vi "S4GUI_003.vi"(7 "Tab ObsEng":enum32{"Obs", "CCD modes", "Guider", "Eng"}(tab)) -> ()   [LabVIEW 2018] (continued)
                        }
                      }
                      frame 3 {
                        n312 = case shown="False" w628 {
                          tunnel: [cluster{u32, u32}[] [{7563008, 7563008}, {7563008, 7563008}] ("Colors [4]") cluster{u32, u32}[] [{16318208, 16318208}, {16318208, 16318208}] ("Colors [4]")] -> w627
                          frame False {
                          }
                          frame True {
                          }
                        }
                        n313 = Not(x=w628) -> (.not. x?=w629:bool)
                      }
                    }
                    "CALW Status" <- w603
                    "PCS" <- w603
                    n314 = property on="CALW Status" class="Bool (strict)"("Colors [4]"=w601) -> ()  [unwired: 2 in, 2 out]
                    n315 = property on="PCS" class="Bool (strict)"("Colors [4]"=w601, "BoolText.Text"=w602) -> ()  [unwired: 2 in, 2 out]
                  }
                  frame #3 {
                    # "ASEL"
                    n316 = Unbundle By Name(w641) -> ("ASEL State"=w640:i32)
                    n317 = Unbundle By Name(w637) -> ("ASEL posname"=w634:string)
                    n318 = local read "ASEL Status"() -> (w635:bool)
                    n319 = case shown="Default" w634 {
                      selector: w634 -> [w642 _ _]
                      tunnel: [w642 "OFF" ("y") "ON" ("y")] -> w633
                      frame Default {
                      }
                      frame "OFF" {
                      }
                      frame "ON" {
                      }
                    }
                    n320 = case shown="3" w640 {
                      tunnel: [cluster{u32, u32}[] [{9868950, 9868950}, {9868950, 9868950}] ("Colors [4]") cluster{u32, u32}[] [{9868950, 9868950}, {9868950, 9868950}] ("Colors [4]") cluster{u32, u32}[] [{16318208, 16318208}, {16318208, 16318208}] ("Colors [4]") cluster{u32, u32}[] [{6618880, 6618880}, {6618880, 6618880}] ("Colors [4]") w660] -> w638
                      tunnel: [FALSE ("WPROT Status") FALSE ("WPROT Status") TRUE FALSE ("WPROT Status") w659] -> w639
                      tunnel: w633 -> [_ _ _ w655 _]
                      tunnel: ["" ("y") "" ("y") "" ("y") w655 "" ("y")] -> w636
                      tunnel: w635 -> [_ _ _ _ w657]
                      frame Default {
                      }
                      frame 0 {
                      }
                      frame 1 {
                      }
                      frame 2 {
                      }
                      frame 3 {
                        n321 = case shown="True" w657 {
                          tunnel: [cluster{u32, u32}[] [{7563008, 7563008}, {7563008, 7563008}] ("Colors [4]") cluster{u32, u32}[] [{16318208, 16318208}, {16318208, 16318208}] ("Colors [4]")] -> w660
                          frame False {
                          }
                          frame True {
                          }
                        }
                        n322 = Not(x=w657) -> (.not. x?=w659:bool)
                      }
                    }
                    "ASEL Status" <- w639
                    "Analyzer" <- w639
                    n323 = property on="Analyzer" class="Bool (strict)"("Colors [4]"=w638, "BoolText.Text"=w636) -> ()  [unwired: 2 in, 2 out]
                    n324 = property on="ASEL Status" class="Bool (strict)"("Colors [4]"=w638) -> ()  [unwired: 2 in, 2 out]
                  }
                  frame #4 {
                    # "GMIR & GFOC"
                    n325 = Unbundle By Name(w670) -> ("GMIR State"=w669:i32, "GFOC State"=w668:i32)
                    n326 = case shown="2" w669 {
                      tunnel: [cluster{u32, u32}[] [{9868950, 9868950}, {9868950, 9868950}] ("Colors [4]") cluster{u32, u32}[] [{9868950, 9868950}, {9868950, 9868950}] ("Colors [4]") cluster{u32, u32}[] [{16318208, 16318208}, {16318208, 16318208}] ("Colors [4]") cluster{u32, u32}[] [{6618880, 6618880}, {6618880, 6618880}] ("Colors [4]") cluster{u32, u32}[] [{16318208, 16318208}, {16318208, 16318208}] ("Colors [4]")] -> w663
                      tunnel: [FALSE ("WPROT Status") FALSE ("WPROT Status") TRUE ("WPROT Status") FALSE ("WPROT Status") TRUE ("WPROT Status")] -> w665
                      frame Default {
                      }
                      frame 0 {
                      }
                      frame 1 {
                      }
                      frame 2 {
                      }
                      frame 3 {
                      }
                    }
                    "GMIR Status" <- w665
                    "GMIR Status 2" <- w665
                    n327 = property on="GMIR Status" class="Bool (strict)"("Colors [4]"=w663) -> ()  [unwired: 2 in, 2 out]
                    n328 = property on="GMIR Status 2" class="Bool (strict)"("Colors [4]"=w663) -> ()  [unwired: 2 in, 2 out]
                    n329 = case shown="Default" w668 {
                      tunnel: [cluster{u32, u32}[] [{9868950, 9868950}, {9868950, 9868950}] ("Colors [4]") cluster{u32, u32}[] [{9868950, 9868950}, {9868950, 9868950}] ("Colors [4]") cluster{u32, u32}[] [{16318208, 16318208}, {16318208, 16318208}] ("Colors [4]") cluster{u32, u32}[] [{6618880, 6618880}, {6618880, 6618880}] ("Colors [4]") cluster{u32, u32}[] [{16318208, 16318208}, {16318208, 16318208}] ("Colors [4]")] -> w664
                      tunnel: [FALSE ("WPROT Status") FALSE ("WPROT Status") TRUE ("WPROT Status") FALSE ("WPROT Status") TRUE ("WPROT Status")] -> w666
                      frame Default {
                      }
                      frame 0 {
                      }
                      frame 1 {
                      }
                      frame 2 {
                      }
                      frame 3 {
                      }
                    }
                    "GFOC Status" <- w666
                    "GFOC Status 2" <- w666
                    n330 = Or(x=w665, y=w666) -> (x .or. y?=w667:bool)
                    n331 = property on="GFOC Status" class="Bool (strict)"("Colors [4]"=w664) -> ()  [unwired: 2 in, 2 out]
                    n332 = property on="GFOC Status 2" class="Bool (strict)"("Colors [4]"=w664) -> ()  [unwired: 2 in, 2 out]
                    n333 = property on="GS led" class="Bool (strict)"("Blinking"=w667, "Value"=w667) -> ()  [unwired: 2 in, 2 out]
                  }
                }
              }
              frame #7 {
                n334 = Unbundle By Name(w693) -> ("Instrument Pos Names"=w692:T21)
                n335 = stacked-sequence {
                  tunnel: w692 -> [w695 w712 w737 w763]
                  tunnel: [_ _ _ w764] -> w691
                  frame #0 {
                    n336 = Unbundle By Name(w695) -> ("WPSEL posname"=w694:string)
                    n337 = case shown="\"L/2\", \"L/4\", \"OFF\"" w694 {
                      selector: w694 -> [_ w696]
                      frame "False", Default {
                      }
                      frame "L/2", "L/4", "OFF" {
                        n338 = First Call?() -> (First Call?: T/F=w697:bool)
                        n339 = case shown="True" w697 {
                          tunnel: w696 -> [_ w698]
                          frame False {
                          }
                          frame True {
                            n340 = case shown="\"False\", Default" w698 {
                              frame "False", Default {
                              }
                              frame "L/2" {
                                w699 = u16 1 items=["OFF", "Lambda/2", "Lambda/4"] ("Lambda Selector")
                                n341 = property on="Lambda Selector" class="Ring (strict)"(error in=errorcluster {"status"=FALSE, "code"=0, "source"=""} ("error in (no error)"), "Value"=w699) -> (error out=w701:errorcluster)  [unwired: 1 in, 1 out]
                                n342 = property on="Lambda Selector" class="Ring (strict)"(error in=w701, "RingText.Text"="Lambda/2" ("Boolean Text.Text")) -> ()  [unwired: 1 in, 2 out]
                              }
                              frame "L/4" {
                                w703 = u16 2 items=["OFF", "Lambda/2", "Lambda/4"] ("Lambda Selector")
                                n343 = property on="Lambda Selector" class="Ring (strict)"(error in=errorcluster {"status"=FALSE, "code"=0, "source"=""} ("error in (no error)"), "Value"=w703) -> (error out=w705:errorcluster)  [unwired: 1 in, 1 out]
                                n344 = property on="Lambda Selector" class="Ring (strict)"(error in=w705, "RingText.Text"="Lambda/4" ("Boolean Text.Text")) -> ()  [unwired: 1 in, 2 out]
                              }
                              frame "OFF" {
                                w708 = u16 0 items=["OFF", "Lambda/2", "Lambda/4"] ("Lambda Selector")
                                (unwired) "Select..." ("Boolean Text.Text")
                                n345 = property on="Lambda Selector" class="Ring (strict)"(error in=errorcluster {"status"=FALSE, "code"=0, "source"=""} ("error in (no error)"), "Value"=w708) -> (error out=w710:errorcluster)  [unwired: 1 in, 1 out]
                                n346 = property on="Lambda Selector" class="Ring (strict)"(error in=w710, "RingText.Text"="OFF" ("Boolean Text.Text")) -> ()  [unwired: 1 in, 2 out]
                              }
                            }
                          }
                        }
                      }
                    }
                  }
                  frame #1 {
                    n347 = Unbundle By Name(w712) -> ("CALW posname"=w711:string)
                    n348 = case shown="\"DEPOLARIZER\", \"OFF\", \"PINHOLE\", \"POLARIZER\", \"SHUTTER\"" w711 {
                      selector: w711 -> [_ w713]
                      frame "False", Default {
                      }
                      frame "DEPOLARIZER", "OFF", "PINHOLE", "POLARIZER", "SHUTTER" {
                        n349 = First Call?() -> (First Call?: T/F=w714:bool)
                        n350 = case shown="True" w714 {
                          tunnel: w713 -> [_ w715]
                          frame False {
                          }
                          frame True {
                            n351 = case shown="\"OFF\"" w715 {
                              frame "False", Default {
                              }
                              frame "POLARIZER" {
                                w716 = u16 1 items=["OFF", "POLARIZER", "PINHOLE", "SHUTTER", "DEPOLARIZER"] ("Calibrator Selector")
                                n352 = property on="Calibrator Selector" class="Ring (strict)"(error in=errorcluster {"status"=FALSE, "code"=0, "source"=""} ("error in (no error)"), "Value"=w716) -> (error out=w718:errorcluster)  [unwired: 1 in, 1 out]
                                n353 = property on="Calibrator Selector" class="Ring (strict)"(error in=w718, "RingText.Text"="POLARIZER" ("Boolean Text.Text")) -> ()  [unwired: 1 in, 2 out]
                              }
                              frame "DEPOLARIZER" {
                                w720 = u16 4 items=["OFF", "POLARIZER", "PINHOLE", "SHUTTER", "DEPOLARIZER"] ("Calibrator Selector")
                                n354 = property on="Calibrator Selector" class="Ring (strict)"(error in=errorcluster {"status"=FALSE, "code"=0, "source"=""} ("error in (no error)"), "Value"=w720) -> (error out=w722:errorcluster)  [unwired: 1 in, 1 out]
                                n355 = property on="Calibrator Selector" class="Ring (strict)"(error in=w722, "RingText.Text"="DEPOLARIZER" ("Boolean Text.Text")) -> ()  [unwired: 1 in, 2 out]
                              }
                              frame "PINHOLE" {
                                w724 = u16 2 items=["OFF", "POLARIZER", "PINHOLE", "SHUTTER", "DEPOLARIZER"] ("Calibrator Selector")
                                n356 = property on="Calibrator Selector" class="Ring (strict)"(error in=errorcluster {"status"=FALSE, "code"=0, "source"=""} ("error in (no error)"), "Value"=w724) -> (error out=w726:errorcluster)  [unwired: 1 in, 1 out]
                                n357 = property on="Calibrator Selector" class="Ring (strict)"(error in=w726, "RingText.Text"="PINHOLE" ("Boolean Text.Text")) -> ()  [unwired: 1 in, 2 out]
                              }
                              frame "SHUTTER" {
                                w728 = u16 3 items=["OFF", "POLARIZER", "PINHOLE", "SHUTTER", "DEPOLARIZER"] ("Calibrator Selector")
                                n358 = property on="Calibrator Selector" class="Ring (strict)"(error in=errorcluster {"status"=FALSE, "code"=0, "source"=""} ("error in (no error)"), "Value"=w728) -> (error out=w730:errorcluster)  [unwired: 1 in, 1 out]
                                n359 = property on="Calibrator Selector" class="Ring (strict)"(error in=w730, "RingText.Text"="SHUTTER" ("Boolean Text.Text")) -> ()  [unwired: 1 in, 2 out]
                              }
                              frame "OFF" {
                                w732 = u16 0 items=["OFF", "POLARIZER", "PINHOLE", "SHUTTER", "DEPOLARIZER"] ("Calibrator Selector")
                                n360 = property on="Calibrator Selector" class="Ring (strict)"(error in=errorcluster {"status"=FALSE, "code"=0, "source"=""} ("error in (no error)"), "Value"=w732) -> (error out=w734:errorcluster)  [unwired: 1 in, 1 out]
                                n361 = property on="Calibrator Selector" class="Ring (strict)"(error in=w734, "RingText.Text"="OFF" ("Boolean Text.Text")) -> ()  [unwired: 1 in, 2 out]
                              }
                            }
                          }
                        }
                      }
                    }
                  }
                  frame #2 {
                    n362 = Unbundle By Name(w737) -> ("WPROT posname"=w736:string)
                    "Name" <- w736
                    n363 = stacked-sequence {
                      tunnel: w736 -> [_ w739]
                      frame #0 {
                        w738 = FALSE
                        "ledP0" <- w738
                        "ledP1" <- w738
                        "ledP2" <- w738
                        "ledP3" <- w738
                        "ledP4" <- w738
                        "ledP5" <- w738
                        "ledP6" <- w738
                        "ledP7" <- w738
                        "ledP8" <- w738
                        "ledP9" <- w738
                        "ledP10" <- w738
                        "ledP11" <- w738
                        "ledP12" <- w738
                        "ledP13" <- w738
                        "ledP14" <- w738
                        "ledP15" <- w738
                      }
                      frame #1 {
                        n364 = case shown="\"WP3\"" w739 {
                          frame Default {
                          }
                          frame "WP1" {
                            n365 = local write "ledP0"(TRUE ("ledP0")) -> ()
                          }
                          frame "WP2" {
                            n366 = local write "ledP1"(TRUE ("ledP0")) -> ()
                          }
                          frame "WP3" {
                            n367 = local write "ledP2"(TRUE ("ledP0")) -> ()
                          }
                          frame "WP4" {
                            n368 = local write "ledP3"(TRUE ("ledP0")) -> ()
                          }
                          frame "WP5" {
                            n369 = local write "ledP4"(TRUE ("ledP0")) -> ()
                          }
                          frame "WP6" {
                            n370 = local write "ledP5"(TRUE ("ledP0")) -> ()
                          }
                          frame "WP7" {
                            n371 = local write "ledP6"(TRUE ("ledP0")) -> ()
                          }
                          frame "WP8" {
                            n372 = local write "ledP7"(TRUE ("ledP0")) -> ()
                          }
                          frame "WP9" {
                            n373 = local write "ledP8"(TRUE ("ledP0")) -> ()
                          }
                          frame "WP10" {
                            n374 = local write "ledP9"(TRUE ("ledP0")) -> ()
                          }
                          frame "WP11" {
                            n375 = local write "ledP10"(TRUE ("ledP0")) -> ()
                          }
                          frame "WP12" {
                            n376 = local write "ledP11"(TRUE ("ledP0")) -> ()
                          }
                          frame "WP13" {
                            n377 = local write "ledP12"(TRUE ("ledP0")) -> ()
                          }
                          frame "WP14" {
                            n378 = local write "ledP13"(TRUE ("ledP0")) -> ()
                          }
                          frame "WP15" {
                            n379 = local write "ledP14"(TRUE ("ledP0")) -> ()
                          }
                          frame "WP16" {
                            n380 = local write "ledP15"(TRUE ("ledP0")) -> ()
                          }
                        }
                      }
                    }
                  }
                  frame #3 {
                    w767 = "OFF" ("Boolean Text.Text")
                    # "Polarimetria:   ASEL = ON  &   (WPSEL =L/2 or L/4)\n\nFotometria:    ASEL=OFF & WPSEL = OFF & CALW = OFF"
                    n381 = Unbundle By Name(w763) -> ("ASEL posname"=w758:string, "WPSEL posname"=w760:string, "CALW posname"=w759:string)
                    n382 = Unbundle By Name(w763) -> ("WPSEL posname"=w770:string, "CALW posname"=w771:string, "ASEL posname"=w765:string)
                    n383 = Equal?(x=w758, y="ON" ("Boolean Text.Text")) -> (x = y?=w761:bool)
                    n384 = case shown="True" w761 {
                      tunnel: w760 -> [w780 w789]
                      tunnel: w759 -> [w779 w783]
                      tunnel: w758 -> [w776 _]
                      tunnel: [FALSE ("Polarimetric Mode") w784] -> w757
                      tunnel: [w772 FALSE ("Photometric Mode")] -> w756
                      frame False {
                        w775 = "OFF" ("Boolean Text.Text")
                        n385 = Equal?(x=w776, y=w775) -> (x = y?=w774:bool)
                        n386 = Equal?(x=w779, y=w775) -> (x = y?=w777:bool)
                        n387 = Equal?(x=w780, y=w775) -> (x = y?=w778:bool)
                        n388 = Compound Arithmetic op=AND(w774, w778, w777) -> (w772:bool)
                      }
                      frame True {
                        n389 = Equal?(x="L/2" ("Boolean Text.Text"), y=w789) -> (x = y?=w790:bool)
                        n390 = Equal?(x="L/4" ("Boolean Text.Text"), y=w789) -> (x = y?=w787:bool)
                        n391 = Not Equal?(x="SHUTTER", y=w783) -> (x != y?=w781:bool)
                        n392 = Or(x=w790, y=w787) -> (x .or. y?=w785:bool)
                        n393 = And(x=w785, y=w781) -> (x .and. y?=w784:bool)
                      }
                    }
                    "Polarimetric Mode" <- w757
                    "Photometric Mode" <- w756
                    n394 = Equal?(x=w767, y=w770) -> (x = y?=w768:bool)
                    n395 = Equal?(x=w767, y=w771) -> (x = y?=w769:bool)
                    n396 = Equal?(x=w767, y=w765) -> (x = y?=w766:bool)
                    n397 = Compound Arithmetic op=AND(w768, w769, w766) -> (invert w764:bool)
                  }
                }
              }
              frame #8 {
                n398 = Unbundle By Name(w796) -> ("ChannelA_Status"=w795:T22, "ChannelB_Status"=w794:T22, "ChannelC_Status"=w792:T22, "ChannelD_Status"=w793:T22)
                n399 = stacked-sequence {
                  tunnel: w795 -> [w884 w940 w992 w1069 _ _ _]
                  tunnel: w794 -> [w883 w938 w991 _ w1090 _ _]
                  tunnel: w793 -> [w881 w935 w989 _ _ _ w1132]
                  tunnel: w792 -> [w882 w936 w990 _ _ w1111 _]
                  frame #0 {
                    n400 = Unbundle By Name(w881) -> ("connection"=w861:bool, "FT"=w843:bool, "Current exp"=w820:dbl, "Cooler ON/OFF"=w875:i16, "Currently temperature"=w872:i16, "Temperature Status"=w869:string, "target  temp"=w805:i16)
                    "Exposure Time ch4" <- w820
                    n401 = Unbundle By Name(w883) -> ("connection"=w863:bool, "FT"=w847:bool, "Current exp"=w831:dbl, "Cooler ON/OFF"=w877:i16, "Currently temperature"=w874:i16, "Temperature Status"=w871:string, "target  temp"=w809:i16)
                    "Exposure Time ch2" <- w831
                    n402 = Unbundle By Name(w884) -> ("connection"=w864:bool, "FT"=w848:bool, "Current exp"=w840:dbl, "Cooler ON/OFF"=w880:i16, "Currently temperature"=w878:i16, "Temperature Status"=w879:string, "target  temp"=w817:i16)
                    "Exposure Time ch1" <- w840
                    n403 = Unbundle By Name(w882) -> ("connection"=w862:bool, "FT"=w845:bool, "Current exp"=w821:dbl, "Cooler ON/OFF"=w876:i16, "Currently temperature"=w873:i16, "Temperature Status"=w870:string, "target  temp"=w806:i16)
                    "Exposure Time ch3" <- w821
                    n404 = Number To Decimal String(number=w805) -> (decimal integer string=→"Target Temp 4":string)  [unwired: 1 in]
                    n405 = Number To Decimal String(number=w806) -> (decimal integer string=→"Target Temp 3":string)  [unwired: 1 in]
                    n406 = Number To Decimal String(number=w809) -> (decimal integer string=→"Target Temp 2":string)  [unwired: 1 in]
                    n407 = Not Equal To 0?(x=w875) -> (x != 0?=w866:bool)
                    n408 = First Call?() -> (First Call?: T/F=w858:bool)
                    n409 = First Call?() -> (First Call?: T/F=w860:bool)
                    n410 = First Call?() -> (First Call?: T/F=w857:bool)
                    n411 = Not Equal To 0?(x=w876) -> (x != 0?=w865:bool)
                    n412 = First Call?() -> (First Call?: T/F=w859:bool)
                    n413 = Number To Decimal String(number=w817) -> (decimal integer string=→"Target Temp 1":string)  [unwired: 1 in]
                    n414 = Number To Fractional String(use system decimal point (T)=FALSE, number=w840, precision (6)=i16 2) -> (F-format string=w837:string)  [unwired: 1 in]
                    n415 = case shown="True" w858 {
                      tunnel: w806 -> [_ w886]
                      frame False {
                      }
                      frame True {
                        n416 = property on="Target Temp 3" class="DigNum (strict)"("Value"=w886) -> ()  [unwired: 2 in, 2 out]
                      }
                    }
                    n417 = case shown="True" w860 {
                      tunnel: w817 -> [_ w888]
                      frame False {
                      }
                      frame True {
                        n418 = property on="Target Temp 1" class="DigNum (strict)"("Value"=w888) -> ()  [unwired: 2 in, 2 out]
                      }
                    }
                    n419 = Number To Fractional String(use system decimal point (T)=FALSE, number=w831, precision (6)=i16 2) -> (F-format string=w832:string)  [unwired: 1 in]
                    n420 = case shown="True" w857 {
                      tunnel: w805 -> [_ w885]
                      frame False {
                      }
                      frame True {
                        n421 = property on="Target Temp 4" class="DigNum (strict)"("Value"=w885) -> ()  [unwired: 2 in, 2 out]
                      }
                    }
                    n422 = Concatenate Strings("Exposure Time ", w837) -> (w836:string)
                    n423 = Number To Fractional String(use system decimal point (T)=FALSE, number=w821, precision (6)=i16 2) -> (F-format string=w822:string)  [unwired: 1 in]
                    n424 = Number To Fractional String(use system decimal point (T)=FALSE, number=w820, precision (6)=i16 2) -> (F-format string=w826:string)  [unwired: 1 in]
                    n425 = Concatenate Strings("Exposure Time ", w832) -> (w830:string)
                    n426 = case shown="True" w859 {
                      tunnel: w809 -> [_ w887]
                      frame False {
                      }
                      frame True {
                        n427 = property on="Target Temp 2" class="DigNum (strict)"("Value"=w887) -> ()  [unwired: 2 in, 2 out]
                      }
                    }
                    n428 = Concatenate Strings("Exposure Time ", w822) -> (w818:string)
                    n429 = Concatenate Strings("Exposure Time ", w826) -> (w819:string)
                    n430 = property on="Exposure Time ch1" class="Slide (strict)"("Caption.Text"=w836) -> ()  [unwired: 2 in, 2 out]
                    n431 = property on="Exposure Time ch2" class="Slide (strict)"("Caption.Text"=w830) -> ()  [unwired: 2 in, 2 out]
                    n432 = property on="Exposure Time ch3" class="Slide (strict)"("Caption.Text"=w818) -> ()  [unwired: 2 in, 2 out]
                    n433 = property on="Exposure Time ch4" class="Slide (strict)"("Caption.Text"=w819) -> ()  [unwired: 2 in, 2 out]
                    n434 = Not Equal To 0?(x=w880) -> (x != 0?=w867:bool)
                    n435 = Not Equal To 0?(x=w877) -> (x != 0?=w868:bool)
                    n436 = case shown="True" w864 {
                      tunnel: w879 -> [_ w919]
                      tunnel: w878 -> [_ w920]
                      tunnel: w867 -> [_ w917]
                      tunnel: [FALSE w917] -> w856
                      tunnel: [i16 0 ("Currently temperature") w920] -> w814
                      tunnel: ["" ("Temperature Status") w919] -> w855
                      tunnel: [FALSE w918] -> w849
                      tunnel: w848 -> [_ w918]
                      frame False {
                      }
                      frame True {
                      }
                    }
                    "Cooler status 1" <- w856
                    "Curr Temp 1" <- w814
                    "Temp Status 1" <- w855
                    "Panel Temp" <- w814
                    "Panel cooler 1" <- w856
                    "FT1" <- w849
                    n437 = case shown="False" w863 {
                      tunnel: w874 -> [_ w911]
                      tunnel: w871 -> [_ w910]
                      tunnel: w868 -> [_ w912]
                      tunnel: [FALSE w912] -> w854
                      tunnel: [i16 0 ("Currently temperature") w911] -> w810
                      tunnel: ["" ("Temperature Status") w910] -> w853
                      tunnel: w847 -> [_ w909]
                      tunnel: [FALSE ("FT") w909] -> w846
                      frame False {
                      }
                      frame True {
                      }
                    }
                    "Panel Temp 2" <- w810
                    "Curr Temp 2" <- w810
                    "Cooler status 2" <- w854
                    "Panel cooler 2" <- w854
                    "Temp Status 2" <- w853
                    "FT2" <- w846
                    n438 = case shown="True" w861 {
                      tunnel: w872 -> [_ w895]
                      tunnel: w869 -> [_ w894]
                      tunnel: w866 -> [_ w896]
                      tunnel: [FALSE w896] -> w851
                      tunnel: [i16 0 ("Currently temperature") w895] -> w798
                      tunnel: ["" ("Temperature Status") w894] -> w850
                      tunnel: w843 -> [_ w893]
                      tunnel: [FALSE ("FT") w893] -> w842
                      frame False {
                      }
                      frame True {
                      }
                    }
                    "Cooler status 4" <- w851
                    "Panel Temp 4" <- w798
                    "Curr Temp 4" <- w798
                    "Temp Status 4" <- w850
                    "Panel cooler 4" <- w851
                    "FT4" <- w842
                    n439 = case shown="True" w862 {
                      tunnel: w873 -> [_ w903]
                      tunnel: w870 -> [_ w902]
                      tunnel: w865 -> [_ w904]
                      tunnel: [FALSE w904] -> w852
                      tunnel: [i16 0 ("Currently temperature") w903] -> w799
                      tunnel: ["" ("Temperature Status") w902] -> w797
                      tunnel: w845 -> [_ w901]
                      tunnel: [FALSE ("FT") w901] -> w844
                      frame False {
                      }
                      frame True {
                      }
                    }
                    "Cooler status 3" <- w852
                    "Panel Temp 3" <- w799
                    "Curr Temp 3" <- w799
                    "Panel cooler 3" <- w852
                    "FT3" <- w844
                    "Temp Status 3" <- w797
                    n440 = Number To Decimal String(number=w810) -> (decimal integer string=w811:string)  [unwired: 1 in]
                    n441 = Number To Decimal String(number=w814) -> (decimal integer string=w815:string)  [unwired: 1 in]
                    n442 = property on="Panel cooler 2" class="Bool (strict)"("BoolText.Text"=w811, "BoolText.Justify"=enum16{"Left", "Center", "Right"}."Right" ("Boolean Text.Justification")) -> ()  [unwired: 2 in, 2 out]
                    n443 = property on="Panel cooler 1" class="Bool (strict)"("BoolText.Text"=w815, "BoolText.Justify"=enum16{"Left", "Center", "Right"}."Right" ("Boolean Text.Justification")) -> ()  [unwired: 2 in, 2 out]
                    n444 = Number To Decimal String(number=w799) -> (decimal integer string=w803:string)  [unwired: 1 in]
                    n445 = Number To Decimal String(number=w798) -> (decimal integer string=w800:string)  [unwired: 1 in]
                    n446 = property on="Panel cooler 3" class="Bool (strict)"("BoolText.Text"=w803, "BoolText.Justify"=enum16{"Left", "Center", "Right"}."Right" ("Boolean Text.Justification")) -> ()  [unwired: 2 in, 2 out]
                    n447 = property on="Panel cooler 4" class="Bool (strict)"("BoolText.Text"=w800, "BoolText.Justify"=enum16{"Left", "Center", "Right"}."Right" ("Boolean Text.Justification")) -> ()  [unwired: 2 in, 2 out]
                  }
                  frame #1 {
                    n448 = Unbundle By Name(w935) -> ("LastFileImage"=→"Last Image ch4":string, "Temperature Status"=w923:string)
                    n449 = Unbundle By Name(w936) -> ("LastFileImage"=→"Last Image ch3":string, "Temperature Status"=w924:string)
                    n450 = Unbundle By Name(w938) -> ("LastFileImage"=→"Last Image ch2":string, "Temperature Status"=w927:string)
                    n451 = Unbundle By Name(w940) -> ("LastFileImage"=→"Last Image ch1":string, "Temperature Status"=w932:string)
                    n452 = case shown="Default" w932 {
                      tunnel: [cluster{u32, u32}[] [{6124107, 6124107}, {6124107, 6124107}] ("Colors [4]") cluster{u32, u32}[] [{6618880, 6618880}, {6618880, 6618880}] ("Colors [4]") cluster{u32, u32}[] [{16318208, 16318208}, {16318208, 16318208}] ("Colors [4]") cluster{u32, u32}[] [{8554752, 8554752}, {8554752, 8554752}] ("Colors [4]")] -> w931
                      tunnel: [FALSE FALSE FALSE TRUE] -> w930
                      frame Default {
                      }
                      frame "TEMPERATURE_STABILIZED" {
                      }
                      frame "TEMPERATURE_NOT_STABILIZED" {
                      }
                      frame "TEMPERATURE_NOT_REACHED" {
                      }
                    }
                    n453 = case shown="\"TEMPERATURE_NOT_REACHED\"" w927 {
                      tunnel: [cluster{u32, u32}[] [{6124107, 6124107}, {6124107, 6124107}] ("Colors [4]") cluster{u32, u32}[] [{6618880, 6618880}, {6618880, 6618880}] ("Colors [4]") cluster{u32, u32}[] [{16318208, 16318208}, {16318208, 16318208}] ("Colors [4]") cluster{u32, u32}[] [{8554752, 8554752}, {8554752, 8554752}] ("Colors [4]")] -> w929
                      tunnel: [FALSE FALSE FALSE TRUE] -> w928
                      frame Default {
                      }
                      frame "TEMPERATURE_STABILIZED" {
                      }
                      frame "TEMPERATURE_NOT_STABILIZED" {
                      }
                      frame "TEMPERATURE_NOT_REACHED" {
                      }
                    }
                    n454 = case shown="\"TEMPERATURE_NOT_REACHED\"" w924 {
                      tunnel: [cluster{u32, u32}[] [{6124107, 6124107}, {6124107, 6124107}] ("Colors [4]") cluster{u32, u32}[] [{6618880, 6618880}, {6618880, 6618880}] ("Colors [4]") cluster{u32, u32}[] [{16318208, 16318208}, {16318208, 16318208}] ("Colors [4]") cluster{u32, u32}[] [{8554752, 8554752}, {8554752, 8554752}] ("Colors [4]")] -> w926
                      tunnel: [FALSE FALSE FALSE TRUE] -> w925
                      frame Default {
                      }
                      frame "TEMPERATURE_STABILIZED" {
                      }
                      frame "TEMPERATURE_NOT_STABILIZED" {
                      }
                      frame "TEMPERATURE_NOT_REACHED" {
                      }
                    }
                    n455 = case shown="\"TEMPERATURE_NOT_REACHED\"" w923 {
                      tunnel: [cluster{u32, u32}[] [{6124107, 6124107}, {6124107, 6124107}] ("Colors [4]") cluster{u32, u32}[] [{6618880, 6618880}, {6618880, 6618880}] ("Colors [4]") cluster{u32, u32}[] [{16318208, 16318208}, {16318208, 16318208}] ("Colors [4]") cluster{u32, u32}[] [{8554752, 8554752}, {8554752, 8554752}] ("Colors [4]")] -> w922
                      tunnel: [FALSE FALSE FALSE TRUE] -> w921
                      frame Default {
                      }
                      frame "TEMPERATURE_STABILIZED" {
                      }
                      frame "TEMPERATURE_NOT_STABILIZED" {
                      }
                      frame "TEMPERATURE_NOT_REACHED" {
                      }
                    }
                    n456 = property on="Cooler status 1" class="Bool (strict)"("Colors [4]"=w931, "Blinking"=w930) -> ()  [unwired: 2 in, 2 out]
                    n457 = property on="Panel cooler 1" class="Bool (strict)"("Colors [4]"=w931, "Blinking"=w930) -> ()  [unwired: 2 in, 2 out]
                    n458 = property on="Cooler status 4" class="Bool (strict)"("Colors [4]"=w922, "Blinking"=w921) -> ()  [unwired: 2 in, 2 out]
                    n459 = property on="Cooler status 3" class="Bool (strict)"("Colors [4]"=w926, "Blinking"=w925) -> ()  [unwired: 2 in, 2 out]
                    n460 = property on="Panel cooler 4" class="Bool (strict)"("Colors [4]"=w922, "Blinking"=w921) -> ()  [unwired: 2 in, 2 out]
                    n461 = property on="Cooler status 2" class="Bool (strict)"("Colors [4]"=w929, "Blinking"=w928) -> ()  [unwired: 2 in, 2 out]
                    n462 = property on="Panel cooler 3" class="Bool (strict)"("Colors [4]"=w926, "Blinking"=w925) -> ()  [unwired: 2 in, 2 out]
                    n463 = property on="Panel cooler 2" class="Bool (strict)"("Colors [4]"=w929, "Blinking"=w928) -> ()  [unwired: 2 in, 2 out]
                  }
                  frame #2 {
                    n464 = Unbundle By Name(w991) -> ("CamStatus"=w984:string, "connection"=w983:bool)
                    n465 = Unbundle By Name(w990) -> ("CamStatus"=w980:string, "connection"=w979:bool)
                    n466 = Unbundle By Name(w989) -> ("CamStatus"=w976:string, "connection"=w975:bool)
                    n467 = Unbundle By Name(w992) -> ("CamStatus"=w988:string, "connection"=w986:bool)
                    n468 = case shown="True" w983 {
                      tunnel: w984 -> [_ w1023]
                      tunnel: [u32 16739417 w1024] -> w981
                      tunnel: ["" ("CamStatus") w1023] -> w982
                      frame False {
                      }
                      frame True {
                        n469 = property on="Acq status string ch2" class="Str"() -> ("Text.BGColor"=w1025:u32)  [unwired: 2 in, 2 out]
                        n470 = case shown="\"\"" w1023 {
                          tunnel: [u32 16688641 w1030 u32 13882323 u32 13882323] -> w1024
                          tunnel: w1025 -> [_ w1029 _ _]
                          frame Default {
                            # "WAITING_EXPOSE_COMMAND"
                          }
                          frame "ACTIVE" {
                            n471 = Equal?(x=w1029, y=u32 16776002) -> (x = y?=w1028:bool)
                            n472 = case shown="False" w1028 {
                              tunnel: [u32 16776002 u32 16449369] -> w1030
                              frame False {
                              }
                              frame True {
                              }
                            }
                          }
                          frame "IDLE" {
                          }
                          frame "" {
                            # "sem resposta do ACS"
                          }
                        }
                      }
                    }
                    "Acq status string ch2" <- w982
                    n473 = case shown="True" w975 {
                      tunnel: w976 -> [_ w995]
                      tunnel: [u32 16739417 w996] -> w973
                      tunnel: ["" ("CamStatus") w995] -> w974
                      frame False {
                      }
                      frame True {
                        n474 = property on="Acq status string ch4" class="Str"() -> ("Text.BGColor"=w997:u32)  [unwired: 2 in, 2 out]
                        n475 = case shown="\"IDLE\"" w995 {
                          tunnel: [u32 16688641 w1002 u32 13882323 u32 13882323] -> w996
                          tunnel: w997 -> [_ w1001 _ _]
                          frame Default {
                            # "WAITING_EXPOSE_COMMAND"
                          }
                          frame "ACTIVE" {
                            n476 = Equal?(x=w1001, y=u32 16776002) -> (x = y?=w1000:bool)
                            n477 = case shown="False" w1000 {
                              tunnel: [u32 16776002 u32 16449369] -> w1002
                              frame False {
                              }
                              frame True {
                              }
                            }
                          }
                          frame "IDLE" {
                          }
                          frame "" {
                            # "sem resposta do ACS"
                          }
                        }
                      }
                    }
                    "Acq status string ch4" <- w974
                    n478 = case shown="True" w979 {
                      tunnel: w980 -> [_ w1009]
                      tunnel: [u32 16739417 w1010] -> w977
                      tunnel: ["" ("CamStatus") w1009] -> w978
                      frame False {
                      }
                      frame True {
                        n479 = property on="Acq status string ch3" class="Str"() -> ("Text.BGColor"=w1011:u32)  [unwired: 2 in, 2 out]
                        n480 = case shown="\"\"" w1009 {
                          tunnel: [u32 16688641 w1016 u32 13882323 u32 13882323] -> w1010
                          tunnel: w1011 -> [_ w1015 _ _]
                          frame Default {
                            # "WAITING_EXPOSE_COMMAND"
                          }
                          frame "ACTIVE" {
                            n481 = Equal?(x=w1015, y=u32 16776002) -> (x = y?=w1014:bool)
                            n482 = case shown="False" w1014 {
                              tunnel: [u32 16776002 u32 16449369] -> w1016
                              frame False {
                              }
                              frame True {
                              }
                            }
                          }
                          frame "IDLE" {
                          }
                          frame "" {
                            # "sem resposta do ACS"
                          }
                        }
                      }
                    }
                    "Acq status string ch3" <- w978
                    n483 = case shown="True" w986 {
                      tunnel: w988 -> [_ w1037]
                      tunnel: [u32 16739417 w1038] -> w987
                      tunnel: ["" ("CamStatus") w1037] -> w985
                      frame False {
                      }
                      frame True {
                        n484 = property on="Acq status string ch1" class="Str"() -> ("Text.BGColor"=w1039:u32)  [unwired: 2 in, 2 out]
                        n485 = case shown="\"\"" w1037 {
                          tunnel: [u32 16688641 w1044 u32 13882323 u32 13882323] -> w1038
                          tunnel: w1039 -> [_ w1043 _ _]
                          frame Default {
                            # "WAITING_EXPOSE_COMMAND"
                          }
                          frame "ACTIVE" {
                            n486 = Equal?(x=w1043, y=u32 16776002) -> (x = y?=w1042:bool)
                            n487 = case shown="False" w1042 {
                              tunnel: [u32 16776002 u32 16449369] -> w1044
                              frame False {
                              }
                              frame True {
                              }
                            }
                          }
                          frame "IDLE" {
                          }
                          frame "" {
                            # "sem resposta do ACS"
                          }
                        }
                      }
                    }
                    "Acq status string ch1" <- w985
                    n488 = property on="Acq status string ch2" class="Str"("Text.BGColor"=w981) -> ()  [unwired: 2 in, 2 out]
                    n489 = property on="Acq status string ch1" class="Str"("Text.BGColor"=w987) -> ()  [unwired: 2 in, 2 out]
                    n490 = property on="Acq status string ch3" class="Str"("Text.BGColor"=w977) -> ()  [unwired: 2 in, 2 out]
                    n491 = property on="Acq status string ch4" class="Str"("Text.BGColor"=w973) -> ()  [unwired: 2 in, 2 out]
                  }
                  frame #3 {
                    w1057 = cluster{u32, u32}[] [{16711680, 16711680}, {15400704, 15400704}, {16776722, 0}, {16776722, 0}]  # amarelo
                    w1056 = cluster{u32, u32}[] [{16711680, 16711680}, {6618880, 6618880}, {16776722, 0}, {16776722, 0}]  # verde
                    # "Se ocupacao do disco maior que\n90%, barra em vermelho."
                    # "Atualiza status CANAL 1"
                    n492 = Unbundle By Name(w1069) -> ("Frames done"=w1066:u32, "connection"=→"Channel 1" →"setupCH1":bool, "conf runing"=w1067:bool, "UsedDisk"=w1051:u16, "operational"=w1054:bool)
                    "Exposures Done ch1" <- w1066
                    "Disk Storage ch1" <- w1051
                    n493 = Number To Decimal String(number=w1066) -> (decimal integer string=w1064:string)  [unwired: 1 in]
                    n494 = Greater?(x=w1051, y=u16 90) -> (0:w1061:bool)
                    n495 = Select(t=u32 16711680, s=w1061, f=u32 16860) -> (s? t:f=w1059:u32)
                    n496 = Concatenate Strings("#Exposures Done ", w1064) -> (w1063:string)
                    n497 = Select(t=w1056, s=w1054, f=w1057) -> (s? t:f=w1055:cluster{u32, u32}[])
                    n498 = property on="setupCH1" class="Bool (strict)"("Blinking"=w1067) -> ()  [unwired: 2 in, 2 out]
                    n499 = property on="Exposures Done ch1" class="Slide (strict)"("Caption.Text"=w1063) -> ()  [unwired: 2 in, 2 out]
                    n500 = property on="Channel 1" class="Bool (strict)"("Colors [4]"=w1055) -> ()  [unwired: 2 in, 2 out]
                    n501 = property on="Disk Storage ch1" class="Slide (strict)"("Fill Color"=w1059) -> ()  [unwired: 2 in, 2 out]
                    n502 = Number To Decimal String(number=w1051) -> (decimal integer string=w1052:string)  [unwired: 1 in]
                    n503 = Concatenate Strings("Disk Storage ", w1052, "%" ("string")) -> (w1050:string)
                    n504 = property on="Disk Storage ch1" class="Slide (strict)"("Caption.Text"=w1050) -> ()  [unwired: 2 in, 2 out]
                  }
                  frame #4 {
                    w1078 = cluster{u32, u32}[] [{16711680, 16711680}, {15400704, 15400704}, {16776722, 0}, {16776722, 0}]  # amarelo
                    w1077 = cluster{u32, u32}[] [{16711680, 16711680}, {6618880, 6618880}, {16776722, 0}, {16776722, 0}]  # verde
                    # "Se ocupacao do disco maior que\n90%, barra em vermelho."
                    # "Atualiza status CANAL 2"
                    n505 = Unbundle By Name(w1090) -> ("Frames done"=w1085:u32, "connection"=→"Channel 2" →"setupCH2":bool, "conf runing"=w1088:bool, "UsedDisk"=w1070:u16, "operational"=w1075:bool)
                    "Exposures Done ch2" <- w1085
                    "Disk Storage ch2" <- w1070
                    n506 = Number To Decimal String(number=w1085) -> (decimal integer string=w1086:string)  [unwired: 1 in]
                    n507 = Greater?(x=w1070, y=u16 90) -> (0:w1082:bool)
                    n508 = Select(t=u32 16711680, s=w1082, f=u32 16860) -> (s? t:f=w1079:u32)
                    n509 = Concatenate Strings("#Exposures Done ", w1086) -> (w1084:string)
                    n510 = Select(t=w1077, s=w1075, f=w1078) -> (s? t:f=w1076:cluster{u32, u32}[])
                    n511 = property on="setupCH2" class="Bool (strict)"("Blinking"=w1088) -> ()  [unwired: 2 in, 2 out]
                    n512 = property on="Disk Storage ch2" class="Slide (strict)"("Fill Color"=w1079) -> ()  [unwired: 2 in, 2 out]
                    n513 = property on="Exposures Done ch2" class="Slide (strict)"("Caption.Text"=w1084) -> ()  [unwired: 2 in, 2 out]
                    n514 = property on="Channel 2" class="Bool (strict)"("Colors [4]"=w1076) -> ()  [unwired: 2 in, 2 out]
                    n515 = Number To Decimal String(number=w1070) -> (decimal integer string=w1073:string)  [unwired: 1 in]
                    n516 = Concatenate Strings("Disk Storage ", w1073, "%" ("string")) -> (w1071:string)
                    n517 = property on="Disk Storage ch2" class="Slide (strict)"("Caption.Text"=w1071) -> ()  [unwired: 2 in, 2 out]
                  }
                  frame #5 {
                    w1099 = cluster{u32, u32}[] [{16711680, 16711680}, {15400704, 15400704}, {16776722, 0}, {16776722, 0}]  # amarelo
                    w1098 = cluster{u32, u32}[] [{16711680, 16711680}, {6618880, 6618880}, {16776722, 0}, {16776722, 0}]  # verde
                    # "Se ocupacao do disco maior que\n90%, barra em vermelho."
                    # "Atualiza status CANAL3"
                    n518 = Unbundle By Name(w1111) -> ("Frames done"=w1106:u32, "connection"=→"Channel 3" →"setupCH3":bool, "conf runing"=w1110:bool, "UsedDisk"=w1092:u16, "operational"=w1097:bool)
                    "Exposures Done ch3" <- w1106
                    "Disk Storage ch3" <- w1092
                    n519 = Number To Decimal String(number=w1106) -> (decimal integer string=w1107:string)  [unwired: 1 in]
                    n520 = Greater?(x=w1092, y=u16 90) -> (0:w1103:bool)
                    n521 = Select(t=u32 16711680, s=w1103, f=u32 16860) -> (s? t:f=w1100:u32)
                    n522 = Concatenate Strings("#Exposures Done ", w1107) -> (w1105:string)
                    n523 = property on="setupCH3" class="Bool (strict)"("Blinking"=w1110) -> ()  [unwired: 2 in, 2 out]
                    n524 = property on="Disk Storage ch3" class="Slide (strict)"("Fill Color"=w1100) -> ()  [unwired: 2 in, 2 out]
                    n525 = Select(t=w1098, s=w1097, f=w1099) -> (s? t:f=w1096:cluster{u32, u32}[])
                    n526 = property on="Exposures Done ch3" class="Slide (strict)"("Caption.Text"=w1105) -> ()  [unwired: 2 in, 2 out]
                    n527 = property on="Channel 3" class="Bool (strict)"("Colors [4]"=w1096) -> ()  [unwired: 2 in, 2 out]
                    n528 = Number To Decimal String(number=w1092) -> (decimal integer string=w1094:string)  [unwired: 1 in]
                    n529 = Concatenate Strings("Disk Storage ", w1094, "%" ("string")) -> (w1091:string)
                    n530 = property on="Disk Storage ch3" class="Slide (strict)"("Caption.Text"=w1091) -> ()  [unwired: 2 in, 2 out]
                  }
                  frame #6 {
                    w1120 = cluster{u32, u32}[] [{16711680, 16711680}, {15400704, 15400704}, {16776722, 0}, {16776722, 0}]  # amarelo
                    w1119 = cluster{u32, u32}[] [{16711680, 16711680}, {6618880, 6618880}, {16776722, 0}, {16776722, 0}]  # verde
                    # "Se ocupacao do disco maior que\n90%, barra em vermelho."
                    # "Atualiza status CANAL4"
                    n531 = Unbundle By Name(w1132) -> ("Frames done"=w1127:u32, "connection"=→"Channel 4" →"setupCH4":bool, "conf runing"=w1131:bool, "UsedDisk"=w1113:u16, "operational"=w1117:bool)
                    "Exposures Done ch4" <- w1127
                    "Disk Storage ch4" <- w1113
                    n532 = Number To Decimal String(number=w1127) -> (decimal integer string=w1128:string)  [unwired: 1 in]
                    n533 = Greater?(x=w1113, y=u16 90) -> (0:w1124:bool)
                    n534 = Select(t=u32 16711680, s=w1124, f=u32 16860) -> (s? t:f=w1121:u32)
                    n535 = Concatenate Strings("#Exposures Done ", w1128) -> (w1126:string)
                    n536 = property on="setupCH4" class="Bool (strict)"("Blinking"=w1131) -> ()  [unwired: 2 in, 2 out]
                    n537 = property on="Disk Storage ch4" class="Slide (strict)"("Fill Color"=w1121) -> ()  [unwired: 2 in, 2 out]
                    n538 = Select(t=w1119, s=w1117, f=w1120) -> (s? t:f=w1118:cluster{u32, u32}[])
                    n539 = property on="Exposures Done ch4" class="Slide (strict)"("Caption.Text"=w1126) -> ()  [unwired: 2 in, 2 out]
                    n540 = property on="Channel 4" class="Bool (strict)"("Colors [4]"=w1118) -> ()  [unwired: 2 in, 2 out]
                    n541 = Number To Decimal String(number=w1113) -> (decimal integer string=w1115:string)  [unwired: 1 in]
                    n542 = Concatenate Strings("Disk Storage ", w1115, "%" ("string")) -> (w1112:string)
                    n543 = property on="Disk Storage ch4" class="Slide (strict)"("Caption.Text"=w1112) -> ()  [unwired: 2 in, 2 out]
                  }
                }
              }
              frame #9 {
                n544 = Unbundle By Name(w1138) -> ("Instrument Status.mode"=w1137:bool)
                n545 = case shown="True" w1137 {
                  tunnel: [0 ("t") w1151] -> w1134
                  tunnel: w1138 -> [_ w1140]
                  frame False {
                    # "Fotometria: #PSD = 0"
                  }
                  frame True {
                    # "Polarimetria: calcula #PSD"
                    n546 = Unbundle By Name(w1140) -> ("WPROT seq"=w1144:u16)
                    n547 = Number To Boolean Array(number=w1144) -> (Boolean array=w1143:bool[])
                    n548 = for {
                      shift-right: [w1155] -> w1146
                      shift-left: 0 -> [w1153]
                      tunnel: w1143 -> [w1152] mode=indexing
                      # "calcula qtd de 1s"
                      n549 = Increment(x=w1153) -> (x+1=w1154:i32)
                      n550 = Select(t=w1154, s=w1152, f=w1153) -> (s? t:f=w1155:i32)
                    }
                    n551 = property on="#Pol. Seq. Done" class="Slide (strict)"() -> ("Scale.Maximum"=w1145:dbl)  [unwired: 2 in, 2 out]
